vi "TIFF Error Ext.vi"(7 "para3":cluster{}, 8 "error in (no error)":errorcluster, 9 "para2":cluster{}, 10 "para1":cluster{}, 11 "para0":u32) -> (0 "error out":errorcluster, 3 "para0 out":u32)   [LabVIEW 2018]
doc: "LIBTIFF_DLL_IMPEXP void TIFFErrorExt(thandle_t, const char*, const char*, ...);"
uses:
  libtiff3.dll
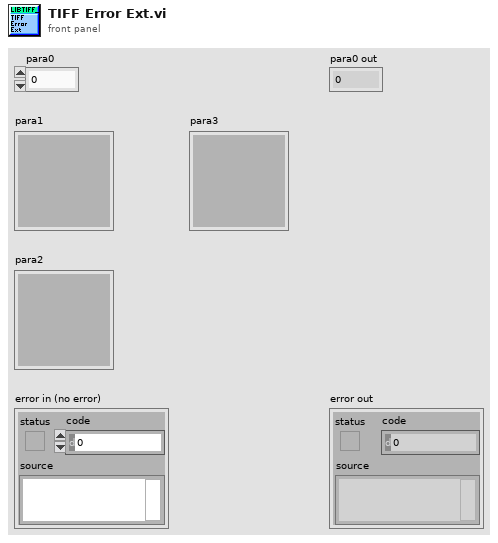
[diagram p1: front panel]
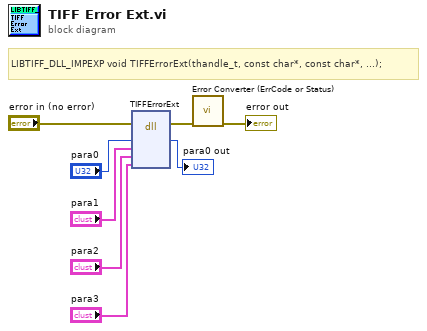
[diagram p0: block diagram]
diagram:
  # "LIBTIFF_DLL_IMPEXP\tvoid TIFFErrorExt(thandle_t, const char*, const char*, ...);"
  n1 = dll-call lib="C:/Users/johan/Downloads/LabVIEW software/LabVIEW software/IX-81 Software/lib/tiff/LibTiffLabview/libtiff3.*" fn="TIFFErrorExt"(error in="error in (no error)", "para0"="para0", "para1"="para1", "para2"="para2", "para3"="para3") -> (error out=w2:errorcluster, "para0"=→"para0 out":u32)  [unwired: 6 in, 1 out]
  n2 = call "Error Converter (ErrCode or Status).vi"("error in (no error)"=w2) -> ("error out"=→"error out":errorcluster)  [unwired: 10 in]
